vi "FGV Spektren automatisch aufzeichnen.vi"(0 "Zeit":u32, 11 "error in (no error)":errorcluster caption="Fehler (Eingang, kein Fehler)", 13 "Aktion":T1) -> (15 "error out":errorcluster caption="Fehler (Ausgang)")   [LabVIEW 2020, in "AK-Schnittstelle.lvlib"]
uses:
  AK-Schnittstelle.lvlib
  Aktion FGV Spektren automatisch aufzeichnen.ctl
  Seiten/FT-IR/FGV FT-IR Aktionen.ctl
  Seiten/FT-IR/FT-IR.lvlib
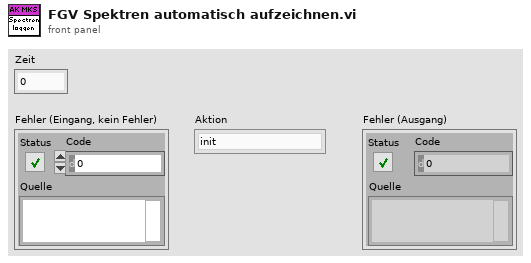
[diagram p1: front panel]
types:
  T1 = typedef "AK-Schnittstelle.lvlib/Aktion FGV Spektren automatisch aufzeichnen.ctl" = enum16{"init", "lesen", "prüfen", "set", "reset"}
  T2 = typedef "FT-IR.lvlib/FGV FT-IR Aktionen.ctl" = enum16{"lesen", "NOG setzen", "NOS setzen", "Initialisieren", "speichern", "ALLES setzen", "FT-IR Spektrum loggen", "Komm Stoppen", "Spektrum LogKonfig"}
  T3 = cluster{"(80) labEnabled":bool, "(81) labPath":path, "(82) labBaseName":string, "(83) labIndex":string, "Spektrum loggen aktiv?":bool}
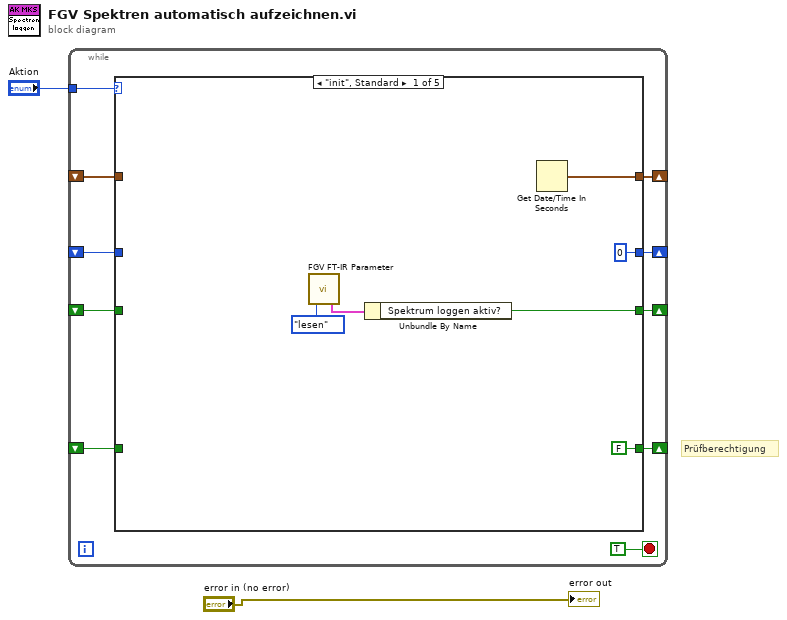
[diagram p0: block diagram]
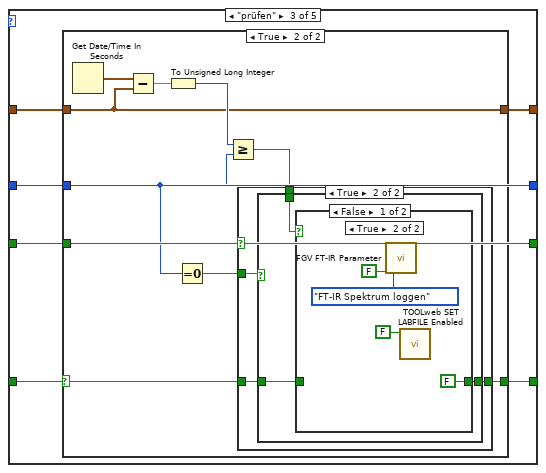
[diagram p3: hidden frame]
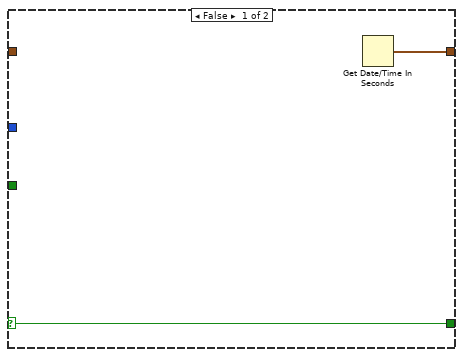
[diagram p4: hidden frame]
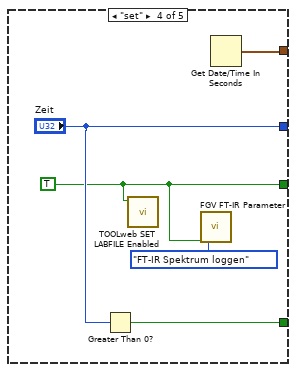
[diagram p8: hidden frame]
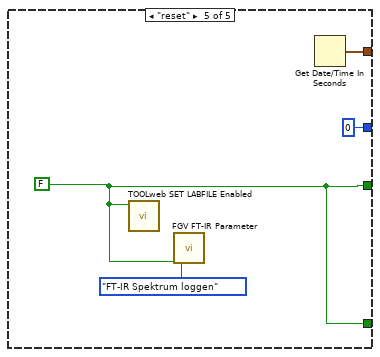
[diagram p9: hidden frame]
diagram:
  # "Prüfberechtigung"
  n1 = while {
    tunnel: "Aktion" -> [w11]
    shift-right: [w10] -> _
    shift-left: _ -> [w9]
    shift-right: [w8] -> _
    shift-left: _ -> [w7]
    shift-right: [w6] -> _
    shift-left: _ -> [w5]
    shift-right: [w4] -> _
    shift-left: _ -> [w3]
    stop <- TRUE stop-if-true
    n2 = case shown="\"init\", Standard" w11 {
      tunnel: [w18 w22 w25 w58 w61] -> w10
      tunnel: w9 -> [_ w22 w26 _ _]
      tunnel: [u32 0 ("Zeit") w21 w28 "Zeit" u32 0 ("Zeit")] -> w8
      tunnel: w7 -> [_ w21 w28 _ _]
      tunnel: [w14 w20 w27 w55 w60] -> w6
      tunnel: w5 -> [_ w20 w27 _ _]
      tunnel: [FALSE ("Spektrum loggen aktiv?") w19 w23 w56 w60] -> w4
      tunnel: w3 -> [_ w19 w24 _ _]
      frame "init", Default {
        n3 = call "FGV FT-IR Parameter.vi"("Aktion"=FGV_FT-IR_Aktionen."lesen") -> ("Ausgangs-Cluster"=w15:T3)  [unwired: 11 in, 7 out]
        n4 = Unbundle By Name(w15) -> ("Spektrum loggen aktiv?"=w14:bool)
        n5 = Get Date/Time In Seconds() -> (seconds since 1Jan1904=w18:timestamp)
      }
      frame "lesen" {
      }
      frame "prüfen" {
        n6 = case shown="True" w24 {
          selector: w24 -> [w29 w32]
          tunnel: w26 -> [_ w33]
          tunnel: w28 -> [_ w36]
          tunnel: w27 -> [_ w35]
          tunnel: [w30 w33] -> w25
          tunnel: [w29 w31] -> w23
          frame False {
            n7 = Get Date/Time In Seconds() -> (seconds since 1Jan1904=w30:timestamp)
          }
          frame True {
            n8 = Get Date/Time In Seconds() -> (seconds since 1Jan1904=w40:timestamp)
            n9 = Subtract(x=w40, y=w33) -> (x-y=w39:dbl)
            n10 = To Unsigned Long Integer(number=w39) -> (unsigned 32bit integer=w34:u32)
            n11 = Equal To 0?(x=w36) -> (x = 0?=w37:bool)
            n12 = Greater Or Equal?(x=w34, y=w36) -> (x >= y?=w38:bool)
            n13 = case shown="True" w35 {
              tunnel: w38 -> [_ w45]
              tunnel: w37 -> [_ w44]
              tunnel: w32 -> [w41 w43]
              tunnel: [w41 w42] -> w31
              frame False {
              }
              frame True {
                n14 = case shown="False" w44 {
                  tunnel: w45 -> [w48 _]
                  tunnel: w43 -> [w47 w54]
                  tunnel: [w46 w54] -> w42
                  frame False {
                    n15 = case shown="True" w48 {
                      tunnel: w47 -> [w49 _]
                      tunnel: [w49 FALSE] -> w46
                      frame False {
                      }
                      frame True {
                        n16 = call "FGV FT-IR Parameter.vi"("Spektrum loggen aktiv?"=FALSE, "Aktion"=FGV_FT-IR_Aktionen."FT-IR Spektrum loggen") -> ()  [unwired: 10 in, 8 out]
                        n17 = call "TOOLweb SET LABFILE Enabled.vi"("Enabled"=FALSE) -> ()  [unwired: 2 in, 5 out]
                      }
                    }
                  }
                  frame True {
                  }
                }
              }
            }
          }
        }
      }
      frame "set" {
        w55 = TRUE ("Spektrum loggen aktiv?")
        n18 = Greater Than 0?(x="Zeit") -> (x > 0?=w56:bool)
        n19 = call "TOOLweb SET LABFILE Enabled.vi"("Enabled"=w55) -> ()  [unwired: 2 in, 5 out]
        n20 = call "FGV FT-IR Parameter.vi"("Spektrum loggen aktiv?"=w55, "Aktion"=FGV_FT-IR_Aktionen."FT-IR Spektrum loggen") -> ()  [unwired: 10 in, 8 out]
        n21 = Get Date/Time In Seconds() -> (seconds since 1Jan1904=w58:timestamp)
      }
      frame "reset" {
        w60 = FALSE ("Spektrum loggen aktiv?")
        n22 = call "TOOLweb SET LABFILE Enabled.vi"("Enabled"=w60) -> ()  [unwired: 2 in, 5 out]
        n23 = call "FGV FT-IR Parameter.vi"("Spektrum loggen aktiv?"=w60, "Aktion"=FGV_FT-IR_Aktionen."FT-IR Spektrum loggen") -> ()  [unwired: 10 in, 8 out]
        n24 = Get Date/Time In Seconds() -> (seconds since 1Jan1904=w61:timestamp)
      }
    }
  }
  "error out" <- "error in (no error)"
